vi "计算类型执行.vi"(8 "error in (no error)":errorcluster caption="错误输入（无错误）", 10 "信号数据":dbl[][](array[numeric]), 11 "计算类型":T1) -> (0 "error out":errorcluster caption="错误输出")   [LabVIEW 2015, in "Logging.lvlib"]
uses:
  Logging.lvlib
  Measure/Measure Type.ctl
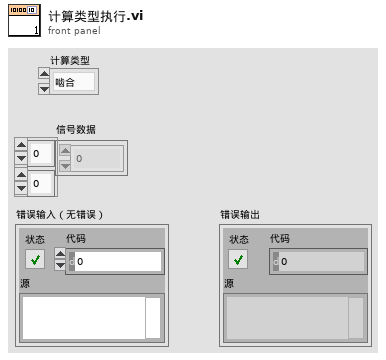
[diagram p1: front panel]
types:
  T1 = typedef "Measure Type.ctl" = enum16{"啮合", "退回", "功能", "力特性", "内泄漏", "分中", "对中"}
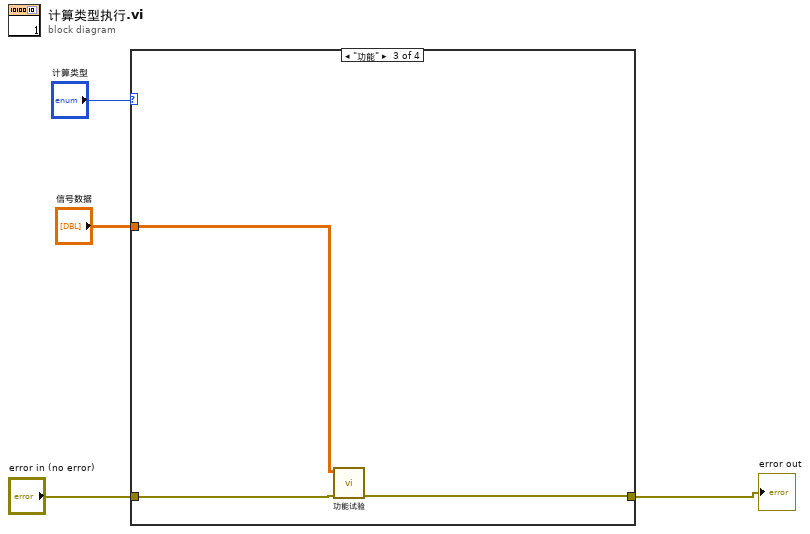
[diagram p0: block diagram]
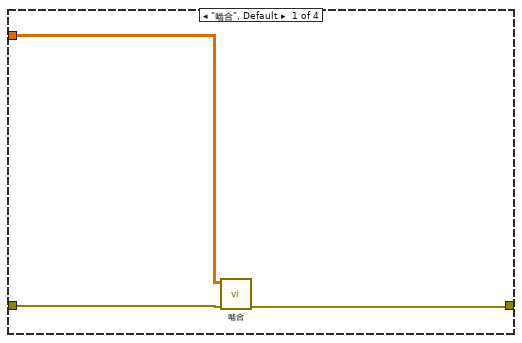
[diagram p2: hidden frame]
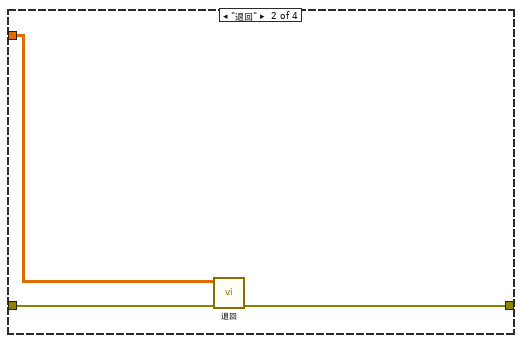
[diagram p3: hidden frame]
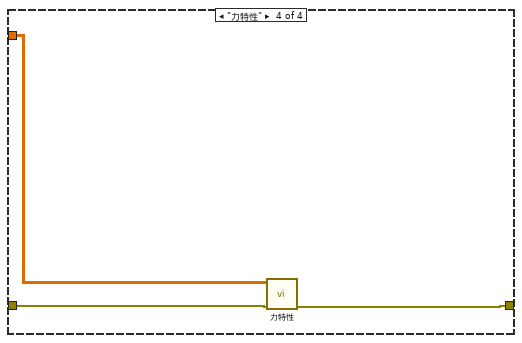
[diagram p4: hidden frame]
diagram:
  n1 = case shown="\"功能\"" "计算类型" {
    tunnel: [w6 w9 w12 w15] -> w3
    tunnel: "error in (no error)" -> [w7 w10 w13 w16]
    tunnel: "信号数据" -> [w5 w8 w11 w14]
    frame "啮合", Default {
      n2 = call "啮合.vi"("error in (no error)"=w7, "信号数据"=w5) -> ("error out"=w6:errorcluster)  [unwired: 9 in]
    }
    frame "退回" {
      n3 = call "退回.vi"("error in (no error)"=w10, "信号数据"=w8) -> ("error out"=w9:errorcluster)  [unwired: 9 in]
    }
    frame "功能" {
      n4 = call "功能试验.vi"("error in (no error)"=w13, "信号数据"=w11) -> ("error out"=w12:errorcluster)  [unwired: 9 in]
    }
    frame "力特性" {
      n5 = call "力特性.vi"("error in (no error)"=w16, "信号数据"=w14) -> ("error out"=w15:errorcluster)  [unwired: 9 in]
    }
  }
  "error out" <- w3
